vi "calibrate_dc_link.vi"(6 "timeout (25000ms)":i32=25000, 8 "error in (no error)":errorcluster, 10 "calibration values":T2, 11 "daemon reference in":refnum<k5>) -> (0 "error out":errorcluster, 1 "response":string, 2 "calibration Result":T1, 3 "daemon reference out":refnum<k5>, 5 "command out":string="random")   [LabVIEW 2017]
doc: "<b>Command: </b>\"calibrate_dc_link\"\n\n<b>Description: </b> This command is to take input from user and calibrate the dc_link gain and offset.\n\n<b>Parameters: </b> adc low & high, measure voltage low & high\n____________________________________________\nDIPC 692 Daemon API 10.0.0.1\nSam Tee - Dyson Technology Ltd\nCopyright (c) 2024, Dyson Technology Ltd"
uses:
  typdef/calibration value.ctl
  typdef/calibration result.ctl
panel:
  out "parameter(s) in":string
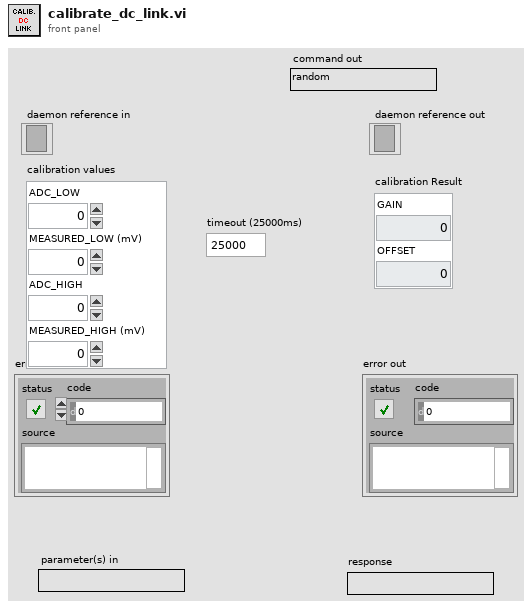
[diagram p1: front panel]
types:
  T1 = typedef "calibration result.ctl" = cluster{"GAIN":dbl, "OFFSET":dbl}
  T2 = typedef "calibration value.ctl" = cluster{"ADC_LOW":dbl, "MEASURED_LOW (mV)":dbl, "ADC_HIGH":dbl, "MEASURED_HIGH (mV)":dbl}
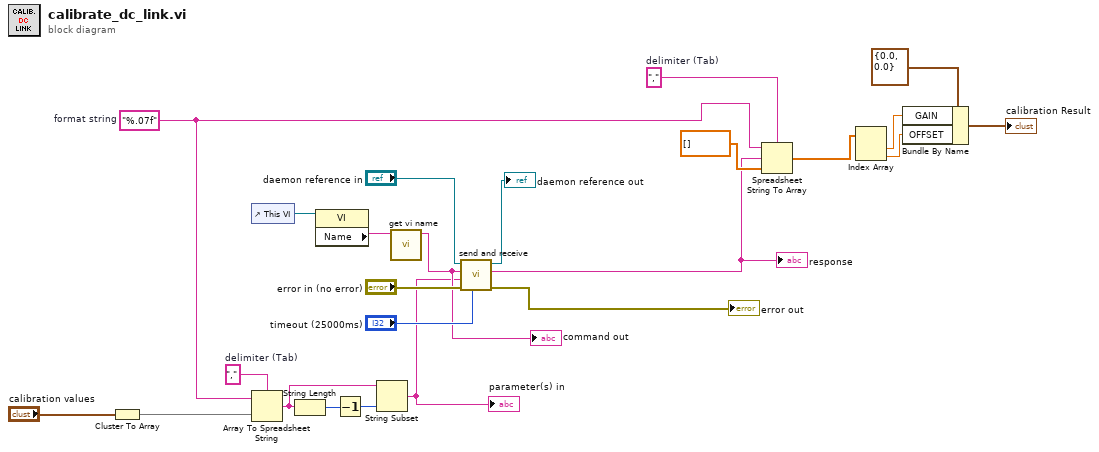
[diagram p0: block diagram]
diagram:
  w2 = "%.07f"  # format string
  w9 = ","  # delimiter (Tab)
  w16 = ","  # delimiter (Tab)
  n1 = Cluster To Array(cluster="calibration values") -> (array=w15:dbl[])
  n2 = control-ref of="This VI"() -> (w19:refnum<vi>)
  n3 = Array To Spreadsheet String(delimiter (Tab)=w16, array=w15, 3:w2) -> (spreadsheet string=w14:string)
  n4 = String Length(string=w14) -> (length=w13:i32)
  n5 = property class="VI"(reference=w19) -> ("Name"=w18:string)  [unwired: 1 in, 2 out]
  n6 = Decrement(x=w13) -> (x-1=w12:i32)
  n7 = String Subset(string=w14, length (rest)=w12) -> (substring=w10:string)  [unwired: 1 in]
  "parameter(s) in" <- w10
  n8 = call "get vi name.vi"("library.lvlib:name.vi"=w18) -> ("vi name"=w17:string)  [unwired: 10 in]
  "command out" <- w17
  n9 = call "send and receive.vi"("timeout (25000ms)"="timeout (25000ms)", "error in (no error)"="error in (no error)", "data"=w10, "command"=w17, "daemon reference in"="daemon reference in") -> ("error out"=→"error out":errorcluster, "response"=w3:string, "daemon reference out"=→"daemon reference out":refnum<k5>)  [unwired: 4 in]
  "response" <- w3
  n10 = Spreadsheet String To Array(delimiter (Tab)=w9, format string=w2, spreadsheet string=w3, array type (2D Dbl)=dbl[] []) -> (array=w1:dbl[])
  n11 = Index Array(array=w1) -> (element #1=w8:dbl, element #2=w7:dbl)  [unwired: 2 in]
  n12 = Bundle By Name(cluster=T1 {"GAIN"=0.0, "OFFSET"=0.0} ("calibration"), "GAIN"=w8, "OFFSET"=w7) -> (→"calibration Result":T1)
